vi "题目2.vi"() -> ()   [LabVIEW 2017]
panel:
  out "数值 2":i32
  out "数值":i32
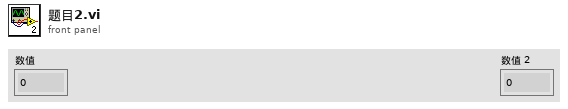
[diagram p1: front panel]
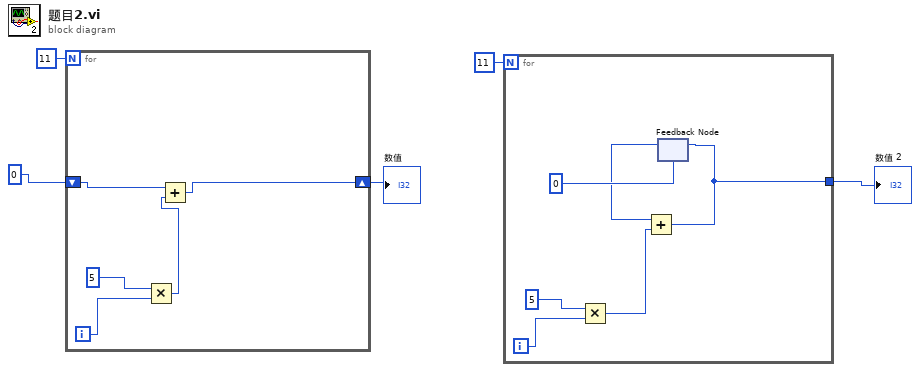
[diagram p0: block diagram]
diagram:
  n1 = for {
    N: 11 -> [_]
    shift-right: [w9] -> w4
    shift-left: 0 -> [w10]
    i -> [w8]
    n2 = Multiply(x=5, y=w8) -> (x*y=w6:i32)
    n3 = Add(x=w10, y=w6) -> (x+y=w9:i32)
  }
  "数值" <- w4
  n4 = for {
    N: 11 -> [_]
    tunnel: [w11] -> w2
    i -> [w14]
    n5 = Multiply(x=5, y=w14) -> (x*y=w12:i32)
    n6 = feedback #1(0) -> (w15:i32)
    n7 = Add(x=w15, y=w12) -> (x+y=w11:i32)
    n8 = feedback-in #1(w11) -> ()
  }
  "数值 2" <- w2
